vi "set_y_resolution.vi"(8 "error in (no error)":errorcluster, 10 "y resolution":i32, 11 "TrajectoryAK101022Resonance in":refnum<class "TrajectoryAK101022Resonance.lvclass">) -> (0 "error out":errorcluster, 3 "TrajectoryAK101022Resonance out":refnum<class "TrajectoryAK101022Resonance.lvclass">)   [LabVIEW 2010, in "TrajectoryAK101022Resonance.lvclass"]
uses:
  TrajectoryAK101022Resonance.lvclass
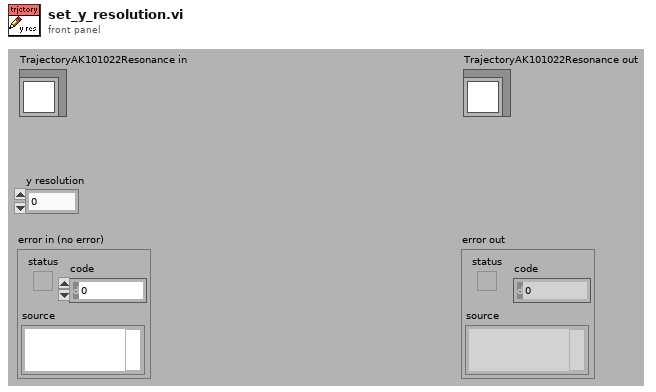
[diagram p1: front panel]
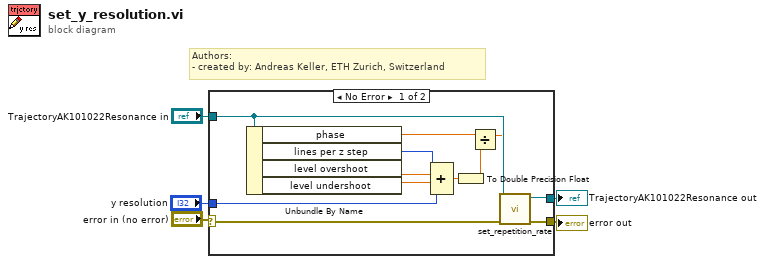
[diagram p0: block diagram]
diagram:
  # "Authors: \n- created by: Andreas Keller, ETH Zurich, Switzerland"
  n1 = case shown="No Error" "error in (no error)" {
    selector: "error in (no error)" -> [w10 w18]
    tunnel: [w9 w18] -> w4
    tunnel: "TrajectoryAK101022Resonance in" -> [w8 w19]
    tunnel: [w7 w19] -> w2
    tunnel: "y resolution" -> [w11 _]
    frame No Error {
      n2 = Unbundle By Name(w8) -> ("phase"=w16:dbl, "lines per z step"=w12:i32, "level overshoot"=w13:dbl, "level undershoot"=w14:dbl)
      n3 = Compound Arithmetic op=ADD(w12, w13, w14, w11) -> (w15:dbl)
      n4 = To Double Precision Float(number=w15) -> (double precision float=w17:dbl)
      n5 = Divide(x=w16, y=w17) -> (x/y=w6:dbl)
      n6 = call-dynamic "set_repetition_rate.vi"("error in (no error)"=w10, "repetition rate"=w6, "TrajectoryAK101022Resonance in"=w8) -> ("error out"=w9:errorcluster, "TrajectoryAK101022Resonance out"=w7:refnum<class "TrajectoryAK101022Resonance.lvclass">)  [unwired: 7 in]
    }
    frame Error {
    }
  }
  "TrajectoryAK101022Resonance out" <- w2
  "error out" <- w4
